vi "Resolution Check.vi"(8 "error in":errorcluster, 9 "new list in":T1[](array[typedef]) {"Last Updated" format="%<%x>T"}, 11 "SR List in":T1[](array[typedef]) {"Last Updated" format="%<%x>T"}) -> (0 "error out":errorcluster, 1 "new list out":T1[](array[typedef]) {"Last Updated" format="%<%x>T"}, 3 "list out":T1[](array[typedef]) {"Last Updated" format="%<%x>T"})   [LabVIEW 2018]
uses:
  SR Status.ctl
  SR Cluster.ctl
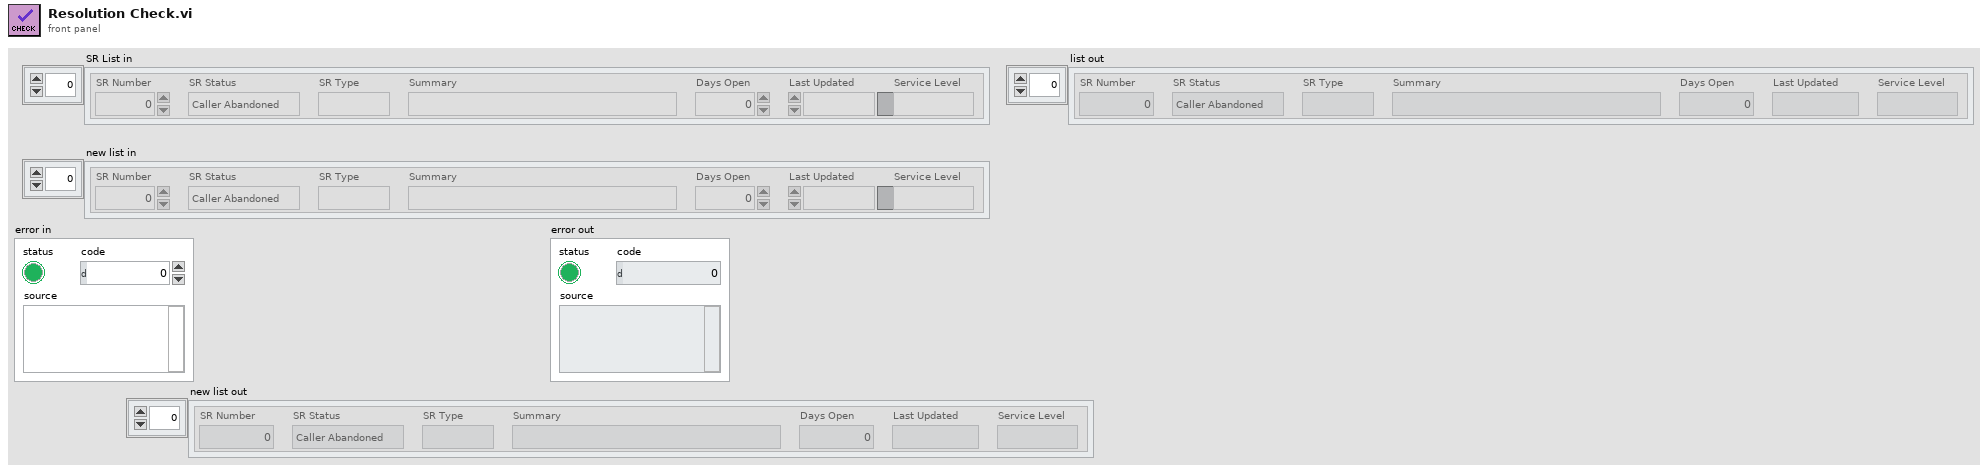
[diagram p1: front panel]
types:
  T1 = typedef "SR Cluster.ctl" = cluster{"SR Number":i32, "SR Type":string, "Summary":string, "Days Open":dbl, "Last Updated":timestamp, "Service Level":string, "SR Status":T2}
  T2 = typedef "SR Status.ctl" = enum16{"Caller Abandoned", "Created in Error", "Expired", "Forum Resolved AE", "Forum Resolved Customer", "IN WORK", "IN WORK Collab with AES", "IN WORK Collab with PSE", "IN WORK Collab with SE", "IN WORK Customer Added Note", "IN WORK Escalation", "IN WORK Wait on Customer", "Open", "Potentially Resolved", "Presumed Resolved", "RMA Approved for Return", "Resolved", "Passed Off"}
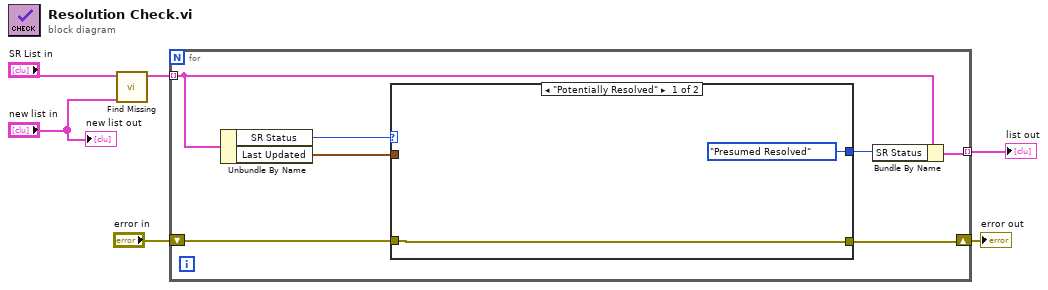
[diagram p0: block diagram]
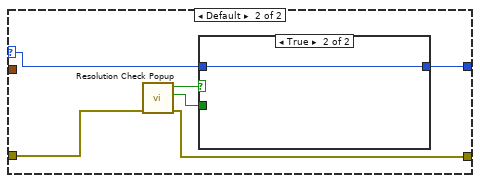
[diagram p2: hidden frame]
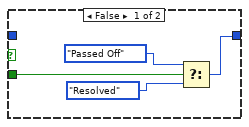
[diagram p3: hidden frame]
diagram:
  n1 = call "Find Missing.vi"("new list in"="new list in", "SR List in"="SR List in") -> ("missing list out"=w4:T1[])  [unwired: 9 in]
  n2 = for {
    tunnel: w4 -> [w10] mode=indexing
    tunnel: [w13] -> w3 mode=indexing
    shift-right: [w8] -> w1
    shift-left: "error in" -> [w9]
    n3 = Unbundle By Name(w10) -> ("SR Status"=w12:T2, "Last Updated"=w11:timestamp)
    n4 = case shown="\"Potentially Resolved\"" w12 {
      selector: w12 -> [_ w19]
      tunnel: w11 -> [_ _]
      tunnel: w9 -> [w15 w18]
      tunnel: [w15 w17] -> w8
      tunnel: [SR_Status."Presumed Resolved" ("SR Status") w16] -> w7
      frame "Potentially Resolved" {
      }
      frame Default {
        n5 = call "Resolution Check Popup.vi"("error in"=w18) -> ("error out"=w17:errorcluster, "Passed Off?"=w21:bool, "Window Closed?"=w20:bool)  [unwired: 8 in]
        n6 = case shown="True" w20 {
          tunnel: [w25 w26] -> w16
          tunnel: w21 -> [w24 _]
          tunnel: w19 -> [_ w26]
          frame False {
            n7 = Select(t=SR_Status."Passed Off" ("SR Status"), s=w24, f=SR_Status."Resolved" ("SR Status")) -> (s? t:f=w25:T2)
          }
          frame True {
          }
        }
      }
    }
    n8 = Bundle By Name(cluster=w10, "SR Status"=w7) -> (w13:T1)
  }
  "list out" <- w3
  "error out" <- w1
  "new list out" <- "new list in"
